vi "Fetch Buffer.vi"(8 "error in (no error)":errorcluster, 9 "Line Number (0)":i32, 10 "Buffer Label (\"Buffer\")":string="Buffer", 11 "VISA resource name":refnum<visa-resource-name>) -> (0 "error out":errorcluster, 2 "Buffer Content":string, 3 "VISA resource name out":refnum<visa-resource-name>)   [LabVIEW 2015, in "Rohde&Schwarz CMXP Base.lvlib"]
doc: "Reads the contents of a buffer line. Buffer contents are stored line by line. Every query generates a new buffer line. The queries are not stored together with the results. Reading buffer contents is non-destructive. The lines can be read in arbitrary order.\n\nAttribute:\n-\n\nRemote-control command:\nFETCh:BASE:BUFFer?"
uses:
  <instrlib>/Rohde&Schwarz CMXP Base/Rohde&Schwarz CMXP Base.lvlib
  <instrlib>/Rohde&Schwarz CMXP Base/Private/rsidr_core.llb/rsidr_core.lvlib
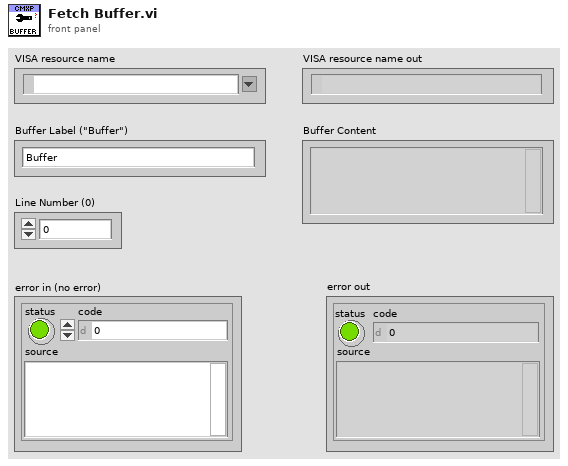
[diagram p1: front panel]
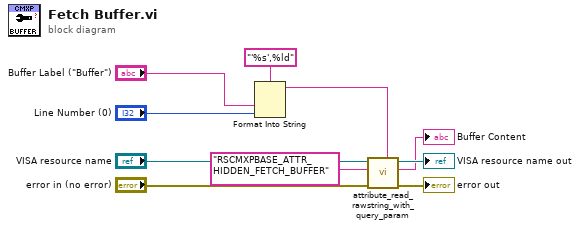
[diagram p0: block diagram]
diagram:
  n1 = Format Into String(format string="'%s',%ld", "Buffer Label (\"Buffer\")", "Line Number (0)") -> (resulting string=w2:string)  [unwired: 2 in, 1 out]
  n2 = call <instrlib>:"attribute_read_rawstring_with_query_param.vi"("Query Parameter (None)"=w2, "error in"="error in (no error)", "Attribute ID"="RSCMXPBASE_ATTR_HIDDEN_FETCH_BUFFER", "VISA resource name"="VISA resource name") -> ("error out"=→"error out":errorcluster, "RawString out"=→"Buffer Content":string, "VISA resource name out"=→"VISA resource name out":refnum<visa-resource-name>)  [unwired: 5 in]
